vi "Generator Lesson 6.vi"() -> ()   [LabVIEW 2019]
uses:
  <vilib>/Instr/_visa.llb/VISA Configure Serial Port (Instr).vi
  <vilib>/addons/control/pid/pid.llb/PID (DBL).vi
  <vilib>/addons/control/pid/NI_PID_pid.lvlib
panel:
  in  "Low":dbl(slide) scale=0.0..200.0
  in  "stop":bool
  out "Meter":dbl(knob) scale=0.0..255.0
  out "Waveform Chart":cluster{dbl, dbl}(graph)
  in  "High":dbl(slide) scale=0.0..200.0
  in  "PID gains":T1={"proportional gain (Kc)"=1.0, "integral time (Ti, min)"=0.01, "derivative time (Td, min)"=0.0} {"derivative time (Td, min)" format="%.3f"; "integral time (Ti, min)" format="%.3f"; "proportional gain (Kc)" format="%.3f"}
  in  "VISA resource name":refnum<visa-resource-name>
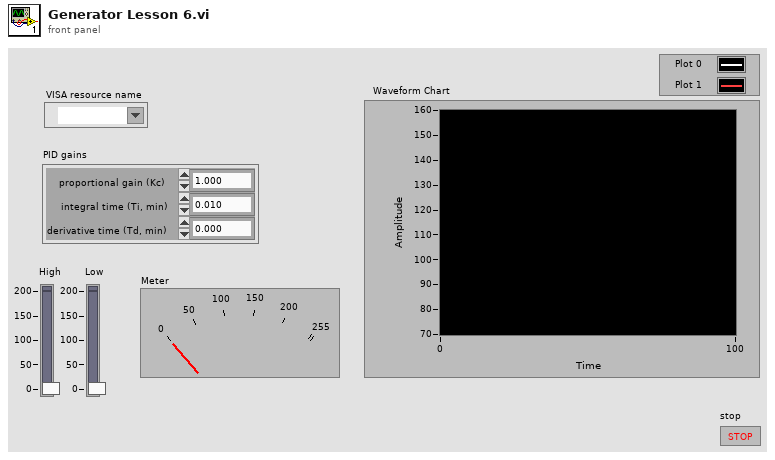
[diagram p1: front panel]
types:
  T1 = cluster{"proportional gain (Kc)":dbl, "integral time (Ti, min)":dbl, "derivative time (Td, min)":dbl}
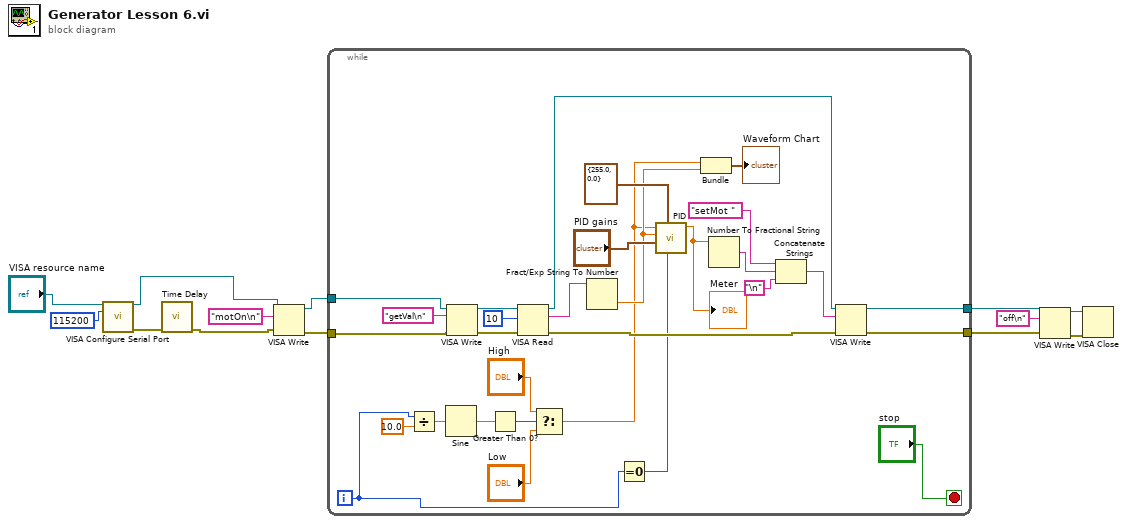
[diagram p0: block diagram]
diagram:
  n1 = call-poly "VISA Configure Serial Port"("VISA resource name"="VISA resource name", "baud rate (9600)"=u32 115200) -> ("VISA resource name out"=w9:refnum<visa-resource-name>, "error out"=w11:errorcluster)  [unwired: 12 in]
  n2 = call "Time Delay"("error in (no error)"=w11) -> ("error out"=w10:errorcluster)  [unwired: 10 in]
  n3 = VISA Write(VISA resource name=w9, write buffer="motOn\n", error in (no error)=w10) -> (VISA resource name out=w7:refnum<visa-resource-name>, error out=w1:errorcluster)  [unwired: 1 out]
  n4 = while {
    tunnel: w7 -> [w24]
    tunnel: w1 -> [w25]
    tunnel: [w32] -> w6
    tunnel: [w31] -> w5
    i -> [w15]
    stop <- "stop" stop-if-true
    n5 = Divide(x=w15, y=sgl 10.0) -> (x/y=w19:sgl)
    n6 = Sine(x=w19) -> (sin(x)=w21:sgl)
    n7 = VISA Write(VISA resource name=w24, write buffer="getVal\n", error in (no error)=w25) -> (VISA resource name out=w43:refnum<visa-resource-name>, error out=w42:errorcluster)  [unwired: 1 out]
    n8 = Greater Than 0?(x=w21) -> (x > 0?=w17:bool)
    n9 = VISA Read(VISA resource name=w43, byte count=u32 10, error in (no error)=w42) -> (VISA resource name out=w33:refnum<visa-resource-name>, read buffer=w41:string, error out=w34:errorcluster)  [unwired: 1 out]
    n10 = Select(t="High", s=w17, f="Low") -> (s? t:f=w22:dbl)
    n11 = Fract/Exp String To Number(string=w41) -> (number=w30:dbl)  [unwired: 3 in, 1 out]
    n12 = Equal To 0?(x=w15) -> (x = 0?=w14:bool)
    n13 = call-poly <vilib>:"PID.vi"("reinitialize? (F)"=w14, "output range"=cluster{"output high":dbl, "output low":dbl} {"output high"=255.0, "output low"=0.0}, "PID gains"="PID gains", "process variable"=w30, "setpoint"=w22) -> ("output"=w28:dbl)  [unwired: 5 in, 1 out]
    "Meter" <- w28
    n14 = Bundle("Low"=w22, w30) -> (→"Waveform Chart":cluster{"Low":dbl, dbl})  [unwired: 1 in]
    n15 = Number To Fractional String(number=w28) -> (F-format string=w37:string)  [unwired: 3 in]
    n16 = Concatenate Strings("setMot " ("string"), w37, "\n") -> (w35:string)
    n17 = VISA Write(VISA resource name=w33, write buffer=w35, error in (no error)=w34) -> (VISA resource name out=w32:refnum<visa-resource-name>, error out=w31:errorcluster)  [unwired: 1 out]
  }
  n18 = VISA Write(VISA resource name=w6, write buffer="off\n", error in (no error)=w5) -> (VISA resource name out=w4:refnum<visa-resource-name>, error out=w3:errorcluster)  [unwired: 1 out]
  n19 = VISA Close(VISA resource name=w4, error in (no error)=w3) -> ()  [unwired: 1 out]
